vi "Post-Build Action.vi"(5 "Files Generated by Build":path[](array[path]), 6 "Top Level/Always Included VIs":path[](array[path]), 7 "Destination Path":path, 8 "error in":errorcluster, 9 "Target Name":string, 10 "Build Specification Name":string, 11 "Project Path":path) -> (0 "error out":errorcluster)   [LabVIEW 2027]
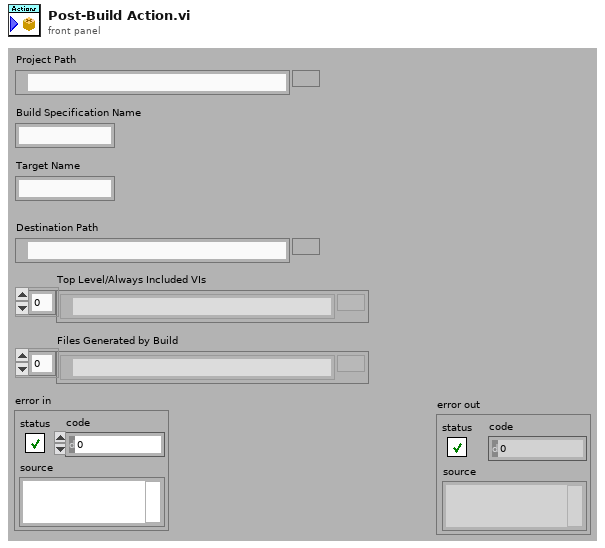
[diagram p1: front panel]
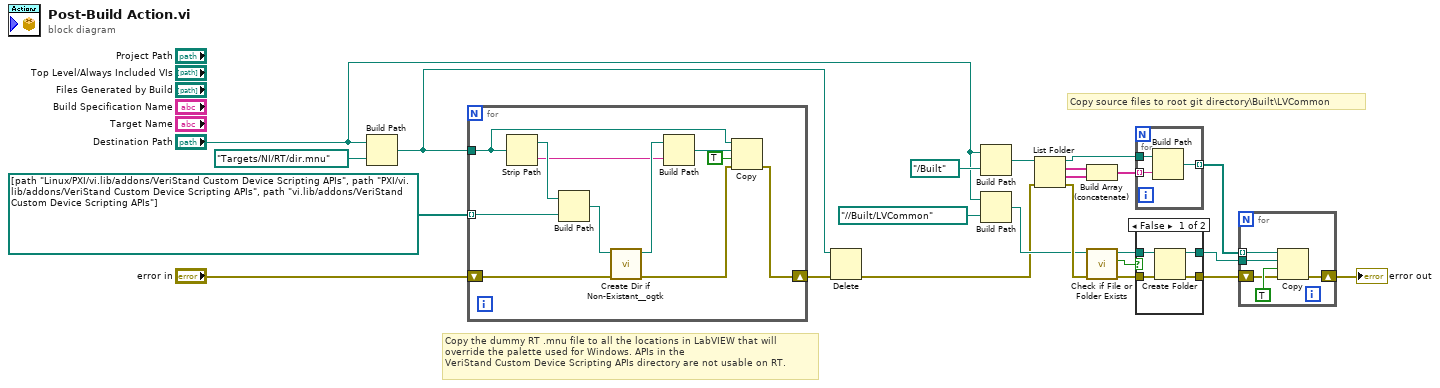
[diagram p0: block diagram]
diagram:
  # "Copy source files to root git directory\\Built\\LVCommon"
  # "Copy the dummy RT .mnu file to all the locations in LabVIEW that will\noverride the palette used for Windows. APIs in the\nVeriStand Custom Device Scripting APIs directory are not usable on RT."
  n1 = Build Path(base path="Destination Path", name or relative path=path "Targets/NI/RT/dir.mnu") -> (appended path=w19:path)
  n2 = for {
    tunnel: w19 -> [w33]
    tunnel: path[] [path "Linux/PXI/vi.lib/addons/VeriStand Custom Device Scripting APIs", path "PXI/vi.lib/addons/VeriStand Custom Device Scripting APIs", path "vi.lib/addons/VeriStand Custom Device Scripting APIs"] -> [w31] mode=indexing
    shift-right: [w26] -> w20
    shift-left: "error in" -> [w25]
    n3 = Strip Path(path=w33) -> (stripped path=w30:path, name=w27:string)
    n4 = Build Path(base path=w30, name or relative path=w31) -> (appended path=w29:path)
    n5 = call <userlib>:"Create Dir if Non-Existant__ogtk.vi"("error in (no error)"=w25, "Directory Path"=w29) -> ("error out"=w24:errorcluster, "dup Directory Path"=w28:path)  [unwired: 7 in, 1 out]
    n6 = Build Path(base path=w28, name or relative path=w27) -> (appended path=w34:path)
    n7 = Copy(8:w24, 9:TRUE ("overwrite (F)"), 10:w34, 11:w33) -> (0:w26:errorcluster)  [unwired: 1 in, 2 out]
  }
  n8 = Delete(path (use dialog)=w19, error in=w20) -> (error out=w3:errorcluster)  [unwired: 3 in, 2 out]
  n9 = Build Path(base path="Destination Path", name or relative path=path "../Built" ("stripped path")) -> (appended path=w11:path)
  n10 = Build Path(base path="Destination Path", name or relative path=path "../../Built/LVCommon" ("stripped path")) -> (appended path=w10:path)
  n11 = List Folder(path=w11, error in=w3) -> (path out=w15:path, filenames=w7:string[], folder names=w6:string[], error out=w14:errorcluster)  [unwired: 2 in]
  n12 = Build Array (concatenate)(w7, w6) -> (w5:string[])
  n13 = call <vilib>:"Check if File or Folder Exists.vi"("error in (no error)"=w14, "path"=w10) -> ("error out"=w16:errorcluster, "file or folder exists?"=w18:bool, "dup path"=w17:path)  [unwired: 7 in]
  n14 = for {
    tunnel: w5 -> [w36] mode=indexing
    tunnel: w15 -> [w37]
    tunnel: [w35] -> w4 mode=indexing
    n15 = Build Path(base path=w37, name or relative path=w36) -> (appended path=w35:path)
  }
  n16 = case shown="False" w18 {
    tunnel: w17 -> [w41 w43]
    tunnel: w16 -> [w40 w42]
    tunnel: [w39 w43] -> w13
    tunnel: [w38 w42] -> w12
    frame False {
      n17 = Create Folder(path (use dialog)=w41, error in=w40) -> (created path=w39:path, error out=w38:errorcluster)  [unwired: 1 in, 1 out]
    }
    frame True {
    }
  }
  n18 = for {
    tunnel: w4 -> [w45] mode=indexing
    shift-right: [w46] -> w2
    shift-left: w12 -> [w47]
    tunnel: w13 -> [w44]
    n19 = Copy(8:w47, 9:TRUE ("overwrite (F)"), 10:w44, 11:w45) -> (0:w46:errorcluster)  [unwired: 1 in, 2 out]
  }
  "error out" <- w2
